vi "delete_password_prompt.vi"(0 "Enable":bool=TRUE, 5 "error in (no error)":errorcluster) -> (17 "password":string, 18 "OK":bool, 19 "error out":errorcluster)   [LabVIEW 2019]
doc: "Displays a standard dialog box that prompts users to enter information, such as a user name and password.\n--------------------\n\nThis Express VI is configured as follows:\n\nMessage to Display to the User:Please input the password for llab_admin\nThe inputs are: \nText Entry Box: password"
panel:
  in  "password":string
  out "String":string="Please input the password for llab_admin"
  in  "OK1":bool
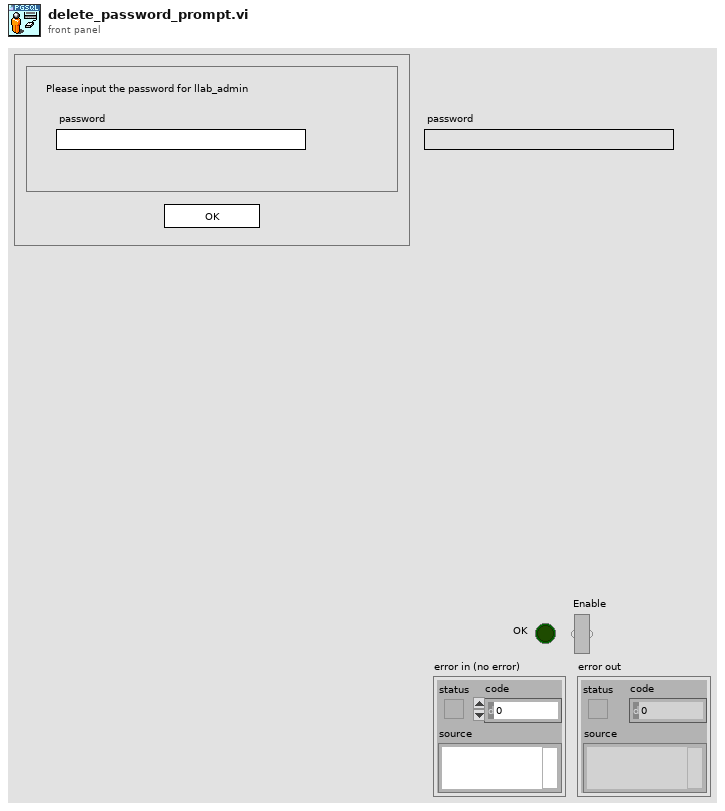
[diagram p1: front panel]
types:
  T1 = cluster{"Input Name":string, "Input Data Type":i32}[]
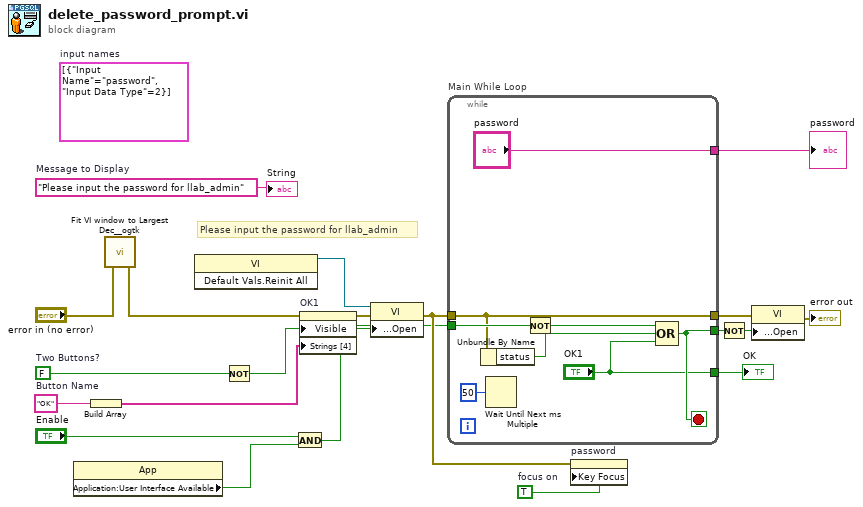
[diagram p0: block diagram]
diagram:
  w5 = TRUE  # focus on
  (unwired) T1 [{"Input Name"="password", "Input Data Type"=2}]  # input names
  w15 = "OK"  # Button Name
  w1 = "Please input the password for llab_admin"  # Message to Display
  w20 = FALSE  # Two Buttons?
  # "Please input the password for llab_admin"
  n1 = property class="App"() -> ("Application:User Interface Available"=w8:bool)  [unwired: 2 in, 2 out]
  n2 = Build Array(w15) -> (w16:string[])
  n3 = call <userlib>:"Fit VI window to Largest Dec__ogtk.vi"("error in (no error)"="error in (no error)") -> ("error out"=w3:errorcluster)  [unwired: 5 in, 1 out]
  n4 = invoke class="VI" method="Default Vals.Reinit All"() -> (reference out=w7:refnum<vi>)  [unwired: 3 in, 2 out]
  n5 = Not(x=w20) -> (.not. x?=w19:bool)
  n6 = And(x="Enable", y=w8) -> (x .and. y?=w9:bool)
  n7 = property on="OK1" class="Bool"(error in=w3, "Visible"=w19, "Strings [4]"=w16) -> (error out=w14:errorcluster)  [unwired: 1 in, 1 out]
  n8 = property class="VI"(reference=w7, error in=w14, "Front Panel Window:Open"=w9) -> (error out=w13:errorcluster)  [unwired: 1 out]
  n9 = while "Main While Loop" {
    tunnel: w9 -> [w27]
    tunnel: [w25] -> w17
    tunnel: w13 -> [w24]
    tunnel: [w24] -> w12
    tunnel: ["password"] -> w6
    tunnel: ["OK1"] -> w2
    stop <- w25 stop-if-true
    n10 = Unbundle By Name(w24) -> ("status"=w23:bool)
    n11 = Wait Until Next ms Multiple(millisecond multiple=u32 50) -> ()  [unwired: 1 out]
    n12 = Not(x=w27) -> (.not. x?=w26:bool)
    n13 = Compound Arithmetic op=OR(w26, w23, "OK1") -> (w25:bool)
  }
  "OK" <- w2
  "password" <- w6
  n14 = property on="password" class="Str"(error in=w13, "Key Focus"=w5) -> ()  [unwired: 1 in, 2 out]
  n15 = Not(x=w17) -> (.not. x?=w18:bool)
  n16 = property class="VI"(error in=w12, "Front Panel Window:Open"=w18) -> (error out=→"error out":errorcluster)  [unwired: 1 in, 1 out]
  "String" <- w1
